vi "Data Inputs.vi"(5 "BBControl Parameters":T1 {"BBControl Criteria"."Comparison" items=["<", ">"]}, 7 "Arm":bool, 8 "error in":errorcluster, 10 "Actuation Array in":bool[](array[boolean]), 11 "Data Notifier":refnum<notifier>) -> (0 "error out":errorcluster, 2 "Actuation Array out":bool[](array[boolean]), 3 "Data Notifier out":refnum<notifier>)   [LabVIEW 2024]
uses:
  support/Control/Array Data Constant.ctl
  support/Control/BBControl Parameters.ctl
  39cb8413-1141-48ba-a68f-b8e0da305499.vi
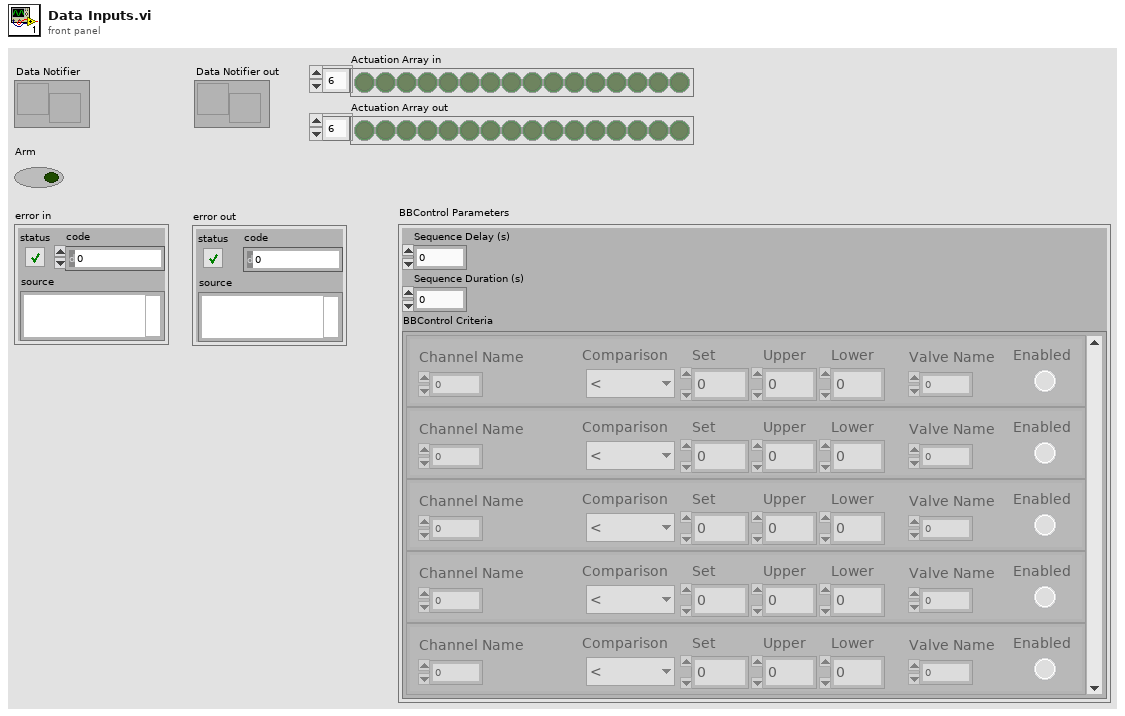
[diagram p1: front panel]
types:
  T1 = typedef "BBControl Parameters.ctl" = cluster{"Sequence Delay (s)":dbl, "Sequence Duration (s)":dbl, "BBControl Criteria":cluster{"Channel Name":i32, "Comparison":u16, "Set":dbl, "Enabled":bool, "Valve Name":i32, "Upper":dbl, "Lower":dbl}[]}
  T2 = cluster{"Channel Name":i32, "Comparison":u16, "Set":dbl, "Enabled":bool, "Valve Name":i32, "Upper":dbl, "Lower":dbl}[]
  T3 = typedef "Array Data Constant.ctl" = cluster{"AI":dbl[], "TC":dbl[], "BC":dbl[], "DI":dbl[], "t (UTC)":dbl}
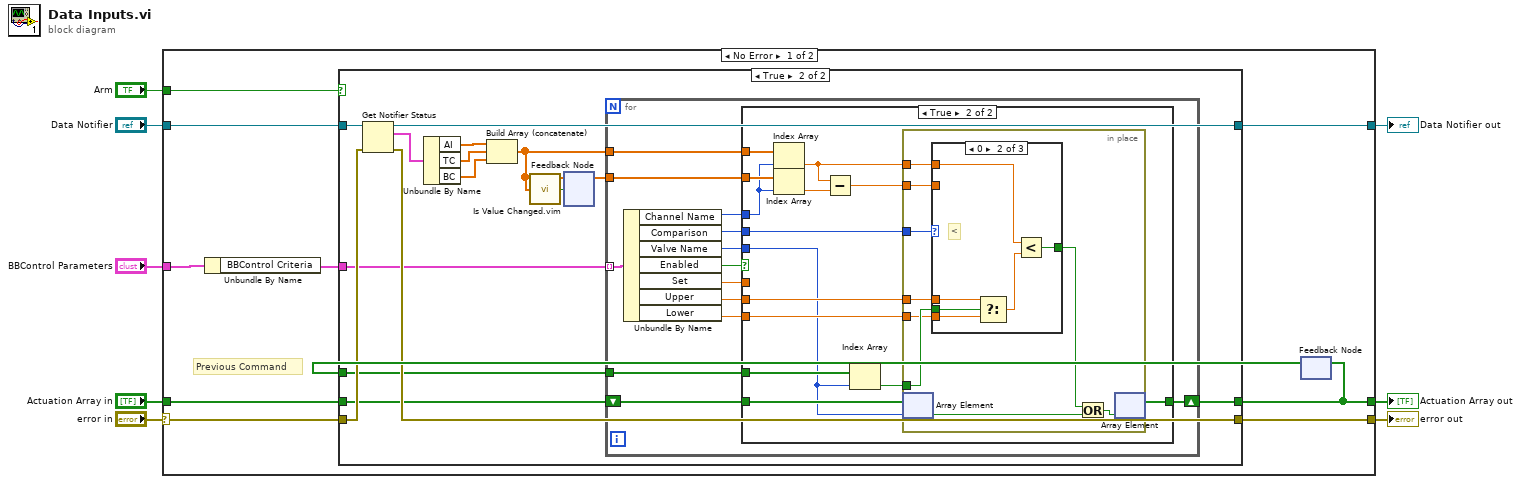
[diagram p0: block diagram]
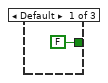
[diagram p4: hidden frame]
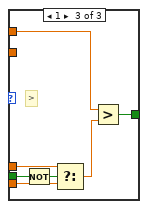
[diagram p5: hidden frame]
diagram:
  n1 = case shown="No Error" "error in" {
    selector: "error in" -> [w16 w89]
    tunnel: [w15 w89] -> w7
    tunnel: "Data Notifier" -> [w18 w90]
    tunnel: [w17 w90] -> w5
    tunnel: "Actuation Array in" -> [w14 w88]
    tunnel: [w10 w88] -> w3
    tunnel: "Arm" -> [w13 _]
    tunnel: "BBControl Parameters" -> [w12 _]
    frame No Error {
      # "Previous Command"
      n2 = Unbundle By Name(w12) -> ("BBControl Criteria"=w11:T2)
      n3 = feedback #1() -> (w9:bool[])  [unwired: 1 in]
      n4 = case shown="True" w13 {
        tunnel: w18 -> [w21 w36]
        tunnel: [w21 w35] -> w17
        tunnel: w16 -> [w19 w34]
        tunnel: [w19 w33] -> w15
        tunnel: w14 -> [w20 w28]
        tunnel: [w20 w27] -> w10
        tunnel: w11 -> [_ w26]
        tunnel: w9 -> [_ w25]
        frame False {
        }
        frame True {
          n5 = Get Notifier Status(notifier=w36, error in (no error)=w34) -> (notifier out=w35:refnum<notifier>, current notification=w32:T3, error out=w33:errorcluster)  [unwired: 2 out]
          n6 = Unbundle By Name(w32) -> ("AI"=w31:dbl[], "TC"=w30:dbl[], "BC"=w29:dbl[])
          n7 = Build Array (concatenate)(w31, w30, w29) -> (w24:dbl[])
          n8 = call "Is Value Changed.vim"("value"=w24) -> ("changed or first call?"=w23:bool)
          n9 = feedback #2() -> (w22:dbl[])  [unwired: 1 in]
          n10 = feedback-in #2(w24, w23) -> ()
          n11 = for {
            tunnel: w26 -> [w47] mode=indexing
            tunnel: w24 -> [w46]
            shift-right: [w48] -> w27
            shift-left: w28 -> [w49]
            tunnel: w25 -> [w38]
            tunnel: w22 -> [w37]
            n12 = Unbundle By Name(w47) -> ("Channel Name"=w43:i32, "Comparison"=w44:u16, "Valve Name"=w45:i32, "Enabled"=w42:bool, "Set"=w41:dbl, "Upper"=w40:dbl, "Lower"=w39:dbl)
            n13 = case shown="True" w42 {
              tunnel: w49 -> [w50 w64]
              tunnel: [w50 w63] -> w48
              tunnel: w46 -> [_ w62]
              tunnel: w45 -> [_ w56]
              tunnel: w44 -> [_ w61]
              tunnel: w43 -> [_ w54]
              tunnel: w41 -> [_ _]
              tunnel: w40 -> [_ w58]
              tunnel: w39 -> [_ w57]
              tunnel: w38 -> [_ w60]
              tunnel: w37 -> [_ w55]
              frame False {
              }
              frame True {
                n14 = Index Array(array=w62, index=w54) -> (element=w52:dbl)
                n15 = Index Array(array=w55, index=w54) -> (element=w53:dbl)
                n16 = Subtract(x=w52, y=w53) -> (x-y=w51:dbl)
                n17 = Index Array(array=w60, index=w56) -> (element=w59:bool)
                n18 = in-place {
                  in-place-border: w61 -> [w71]
                  in-place-border: w52 -> [w70]
                  in-place-border: w59 -> [w69]
                  in-place-border: w58 -> [w68]
                  in-place-border: w57 -> [w67]
                  in-place-border: w51 -> [w65]
                  n19 = in-place-array #3(w64, w56) -> (w72:bool)
                  n20 = case shown="0" w71 {
                    tunnel: w70 -> [_ w80 w87]
                    tunnel: w69 -> [_ w77 w84]
                    tunnel: w68 -> [_ w79 w86]
                    tunnel: w67 -> [_ w78 w85]
                    tunnel: [FALSE w75 w82] -> w66
                    tunnel: w65 -> [_ _ _]
                    frame Default {
                    }
                    frame 0 {
                      # "<"
                      n21 = Select(t=w79, s=w77, f=w78) -> (s? t:f=w76:dbl)
                      n22 = Less?(x=w80, y=w76) -> (x < y?=w75:bool)
                    }
                    frame 1 {
                      # ">"
                      n23 = Not(x=w84) -> (.not. x?=w81:bool)
                      n24 = Select(t=w86, s=w81, f=w85) -> (s? t:f=w83:dbl)
                      n25 = Greater?(x=w87, y=w83) -> (0:w82:bool)
                    }
                  }
                  n26 = Or(x=w66, y=w72) -> (x .or. y?=w73:bool)
                  n27 = in-place-array #3(w73) -> (w63:bool[])  [unwired: 1 out]
                }
              }
            }
          }
        }
      }
      n28 = feedback-in #1(w10) -> ()
    }
    frame Error {
    }
  }
  "Data Notifier out" <- w5
  "error out" <- w7
  "Actuation Array out" <- w3
